vi "Find V1-V2 Interval (SubVI).vi"(9 "V2":i16, 10 "V1":i16, 11 "N Points":i16) -> (2 "V2-V1":i16, 3 "V1-V2":i16)   [LabVIEW 2015]
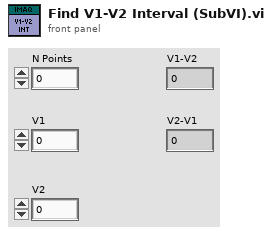
[diagram p1: front panel]
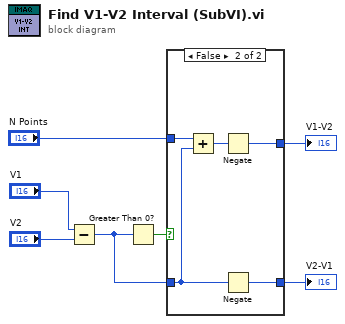
[diagram p0: block diagram]
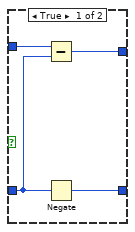
[diagram p2: hidden frame]
diagram:
  n1 = Subtract(x="V1", y="V2") -> (x-y=w4:i16)
  n2 = Greater Than 0?(x=w4) -> (x > 0?=w6:bool)
  n3 = case shown="False" w6 {
    tunnel: "N Points" -> [w8 w13]
    tunnel: w4 -> [w11 w16]
    tunnel: [w10 w15] -> w1
    tunnel: [w9 w14] -> w2
    frame True {
      n4 = Subtract(x=w8, y=w11) -> (x-y=w9:i16)
      n5 = Negate(x=w11) -> (-x=w10:i16)
    }
    frame False {
      n6 = Add(x=w13, y=w16) -> (x+y=w12:i16)
      n7 = Negate(x=w12) -> (-x=w14:i16)
      n8 = Negate(x=w16) -> (-x=w15:i16)
    }
  }
  "V1-V2" <- w2
  "V2-V1" <- w1
